vi "Model 3566-Release.vi"(8 "error in":errorcluster, 11 "Model 3566 Setting":T1) -> (0 "error out":errorcluster)   [LabVIEW 2018]
uses:
  Data Def/Model 3566-Setting.ctl
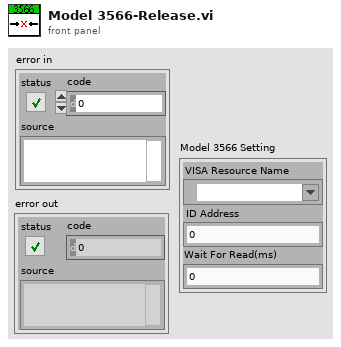
[diagram p1: front panel]
types:
  T1 = typedef "Model 3566-Setting.ctl" = cluster{"VISA Resource Name":refnum<visa-resource-name>, "ID Address":u8, "Wait For Read(ms)":u32}
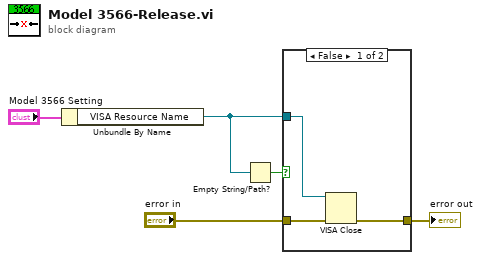
[diagram p0: block diagram]
diagram:
  n1 = Unbundle By Name("Model 3566 Setting") -> ("VISA Resource Name"=w1:refnum<visa-resource-name>)
  n2 = Empty String/Path?(string/path=w1) -> (empty?=w5:bool)
  n3 = case shown="False" w5 {
    tunnel: w1 -> [w7 _]
    tunnel: "error in" -> [w8 w9]
    tunnel: [w6 w9] -> w3
    frame False {
      n4 = VISA Close(VISA resource name=w7, error in (no error)=w8) -> (error out=w6:errorcluster)
    }
    frame True {
    }
  }
  "error out" <- w3
